vi "Write Sequence Call Step.vi"(8 "error in (no error)":errorcluster, 10 "Cluster":T1, 11 "Generic DUT Setup in":refnum<class "Generic DUT Setup.lvclass">) -> (0 "error out":errorcluster, 3 "Generic DUT Setup out":refnum<class "Generic DUT Setup.lvclass">)   [LabVIEW 2018, in "Generic DUT Setup.lvlib" / "Generic DUT Setup.lvclass"]
uses:
  Generic DUT Setup.lvclass
  Plugins/Sequence Call Step Dictionary.lvlibp/Controls/Sequence Call Step.ctl
  Plugins/Sequence Call Step Dictionary.lvlibp/Controls/Parameter.ctl
  Generic DUT Setup.lvclass/Generic DUT Setup.ctl
  Plugins/Sequence Call Step Dictionary.lvlibp/Sequence Call Step Dictionary.lvclass
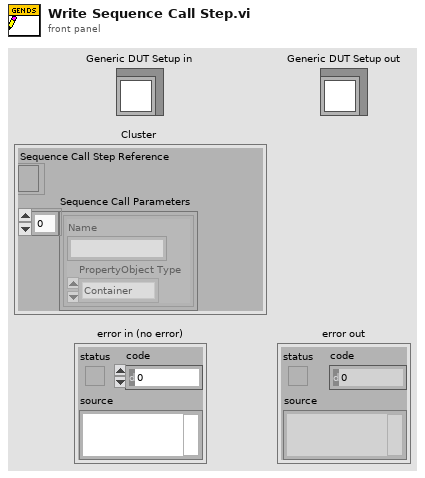
[diagram p1: front panel]
types:
  T1 = typedef "Sequence Call Step Dictionary.lvlibp/Sequence Call Step Dictionary.lvclass/Sequence Call Step.ctl" = cluster{"Sequence Call Step Reference":refnum<k7>, "Sequence Call Parameters":T2[]}
  T2 = typedef "Sequence Call Step Dictionary.lvlibp/Sequence Call Step Dictionary.lvclass/Parameter.ctl" = cluster{"Name":string, "PropertyObject Type":enum16{"Container", "String", "Boolean", "Number", "NamedType", "Reference", "Array", "Aperture Time"}}
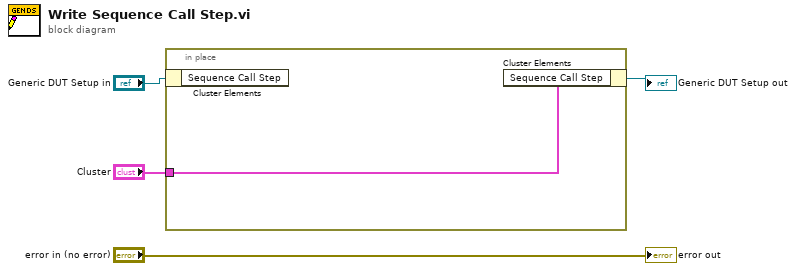
[diagram p0: block diagram]
diagram:
  n1 = in-place {
    in-place-border: "Cluster" -> [w5]
    n2 = in-place-cluster #1("Generic DUT Setup in") -> ()  [unwired: 1 out]
    n3 = in-place-cluster #1("Sequence Call Step"=w5) -> (→"Generic DUT Setup out":refnum<class "Generic DUT Setup.lvclass">)
  }
  "error out" <- "error in (no error)"
